vi "Save Data_IIT.vi"(0 "Experiment Indicator":string, 3 "Scan direction":i32, 4 "Data Array":dbl[][](array[numeric]), 6 "Username":string, 7 "Stabilisation time (ms)":dbl, 8 "Cell details cluster":T1={"Cell Position"=16, "Cell Label"="", "Pixel to measure"=0, "Area (cm^2)"=0.126, "Variable"="", "Variable value"="", "Scan settings in queue"=0, "Light or dark"="", "Measurement Type"=""} {"Pixel to measure" items=["All", "1", "2", "3", "4", "5", "6", "7", "8"]}, 10 "Measurement Delay (ms)":dbl=1.0, 11 "Stabilisation level \n(A or V depending on mode)":dbl=-1.4, 13 "Stabilisation Data":dbl[][](array[numeric])) -> (14 "Master Log":string[][](table), 15 "File path for master log":path, 17 "File path for JV data":path, 18 "File path for JV image":path)   [LabVIEW 2011]
uses:
  <vilib>/Utility/file.llb/Write To Spreadsheet File (string).vi
  <vilib>/Utility/file.llb/Read From Spreadsheet File (string).vi
  <vilib>/Analysis/NI_AALPro.lvlib
panel:
  out "Vmp":dbl
  out "PCE":dbl
  out "FF":dbl
  out "Voc":dbl
  out "Jsc":dbl
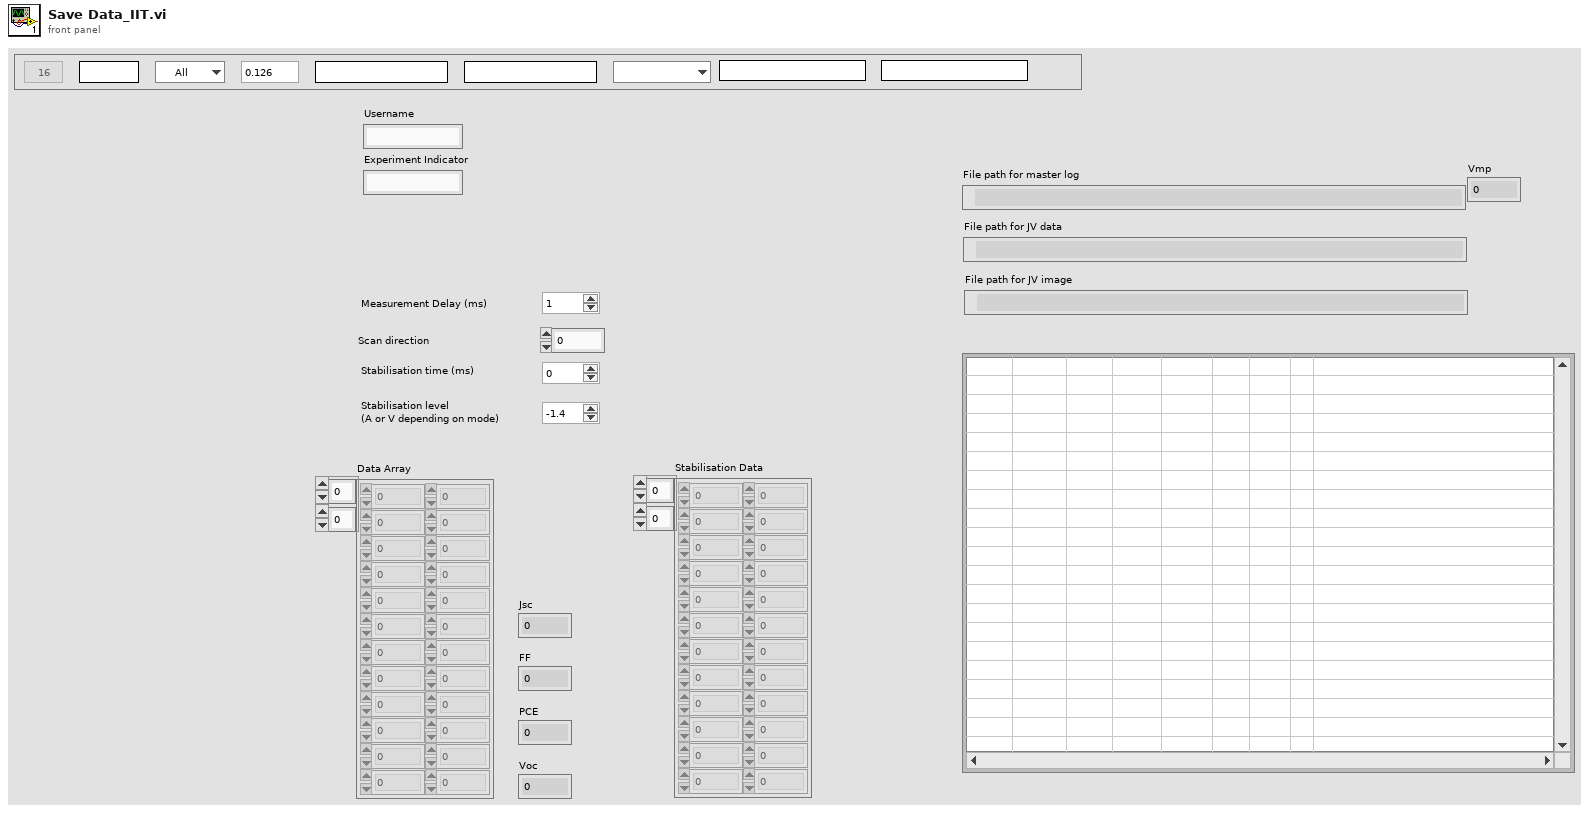
[diagram p1: front panel]
types:
  T1 = cluster{"Cell Position":i32, "Cell Label":string, "Pixel to measure":u16, "Area (cm^2)":dbl, "Variable":string, "Variable value":string, "Scan settings in queue":u16, "Light or dark":string, "Measurement Type":string}
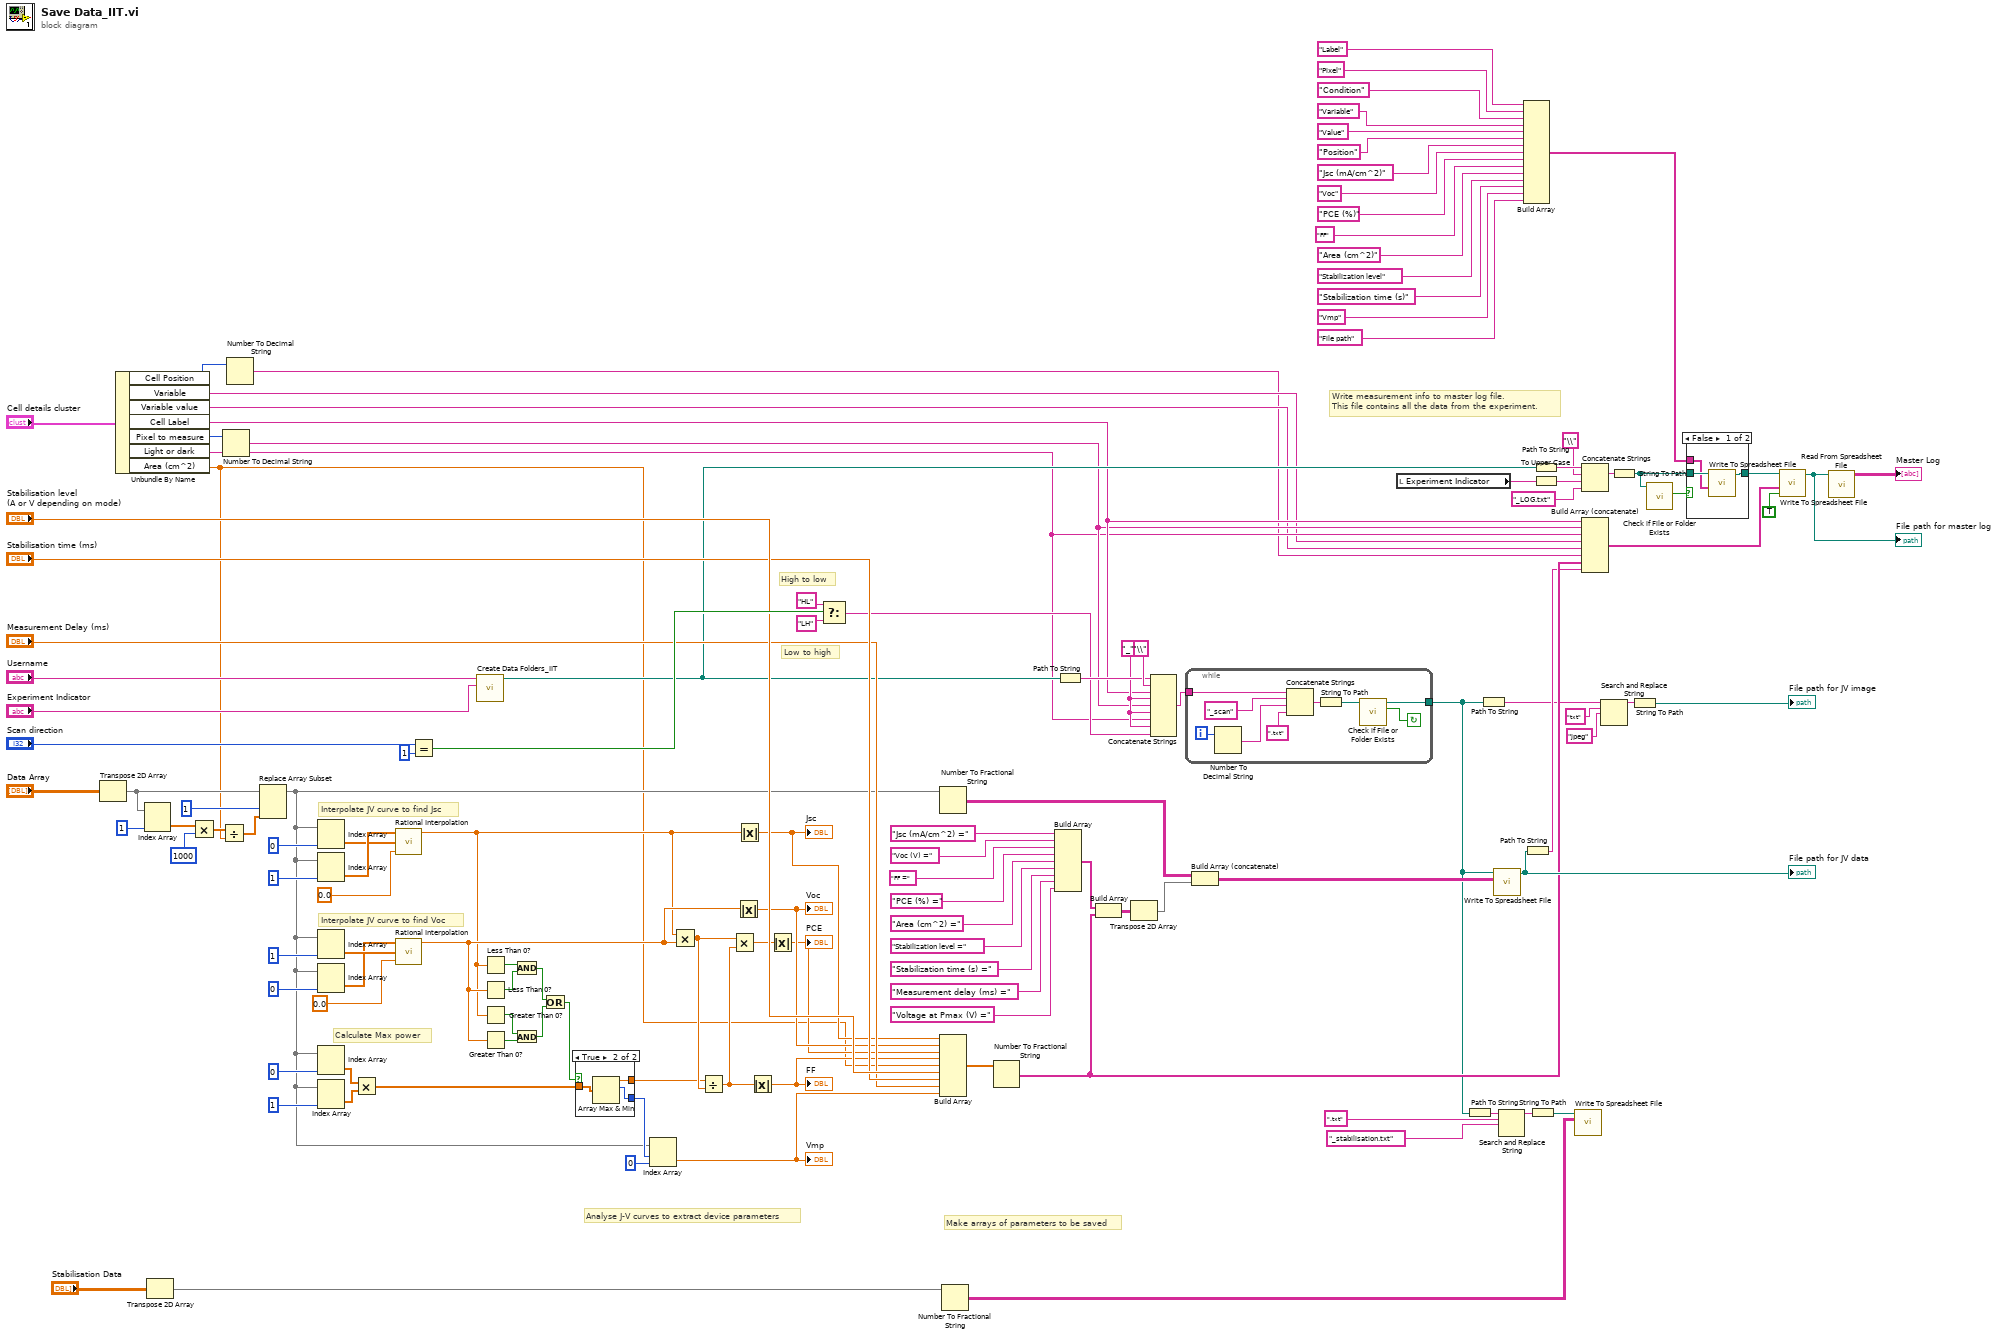
[diagram p0: block diagram]
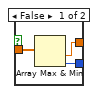
[diagram p3: hidden frame]
diagram:
  w45 = "_"
  # "Make arrays of parameters to be saved"
  # "Calculate Max power"
  # "Interpolate JV curve to find Voc"
  # "Interpolate JV curve to find Jsc"
  # "Analyse J-V curves to extract device parameters"
  # "Write measurement info to master log file.\nThis file contains all the data from the experiment."
  # "Low to high"
  # "High to low"
  n1 = Transpose 2D Array(2D array="Data Array") -> (transposed array=w53:dbl[][])
  n2 = Unbundle By Name("Cell details cluster") -> ("Cell Position"=w26:i32, "Variable"=w22:string, "Variable value"=w21:string, "Cell Label"=w25:string, "Pixel to measure"=w27:u16, "Light or dark"=w23:string, "Area (cm^2)"=w28:dbl)
  n3 = Index Array(array=w53, index (col)=1) -> (element=w51:dbl[])  [unwired: 1 in]
  n4 = Transpose 2D Array(2D array="Stabilisation Data") -> (transposed array=w35:dbl[][])
  n5 = Multiply(x=w51, y=1000) -> (x*y=w48:dbl[])
  n6 = Divide(x=w48, y=w28) -> (x/y=w47:dbl[])
  n7 = Number To Decimal String(number=w27) -> (decimal integer string=w24:string)  [unwired: 1 in]
  n8 = Number To Decimal String(number=w26) -> (decimal integer string=w20:string)  [unwired: 1 in]
  n9 = Replace Array Subset(array=w53, new element=w47, index (col)=1) -> (w32:dbl[][])  [unwired: 1 in]
  n10 = Index Array(array=w32, index (col)=0) -> (element=w120:dbl[])  [unwired: 1 in]
  n11 = Index Array(array=w32, index (col)=1) -> (element=w121:dbl[])  [unwired: 1 in]
  n12 = Index Array(array=w32, index (col)=1) -> (element=w119:dbl[])  [unwired: 1 in]
  n13 = Index Array(array=w32, index (col)=0) -> (element=w117:dbl[])  [unwired: 1 in]
  n14 = Index Array(array=w32, index (col)=0) -> (element=w125:dbl[])  [unwired: 1 in]
  n15 = Index Array(array=w32, index (col)=1) -> (element=w124:dbl[])  [unwired: 1 in]
  n16 = Multiply(x=w125, y=w124) -> (x*y=w118:dbl[])
  n17 = call <vilib>:"Rational Interpolation.vi"("x value"=0.0, "X"=w120, "Y"=w121) -> ("interpolation value"=w49:dbl)  [unwired: 2 out]
  n18 = call <vilib>:"Rational Interpolation.vi"("x value"=0.0, "X"=w119, "Y"=w117) -> ("interpolation value"=w60:dbl)  [unwired: 2 out]
  n19 = Equal?(x="Scan direction", y=1) -> (x = y?=w84:bool)
  n20 = call "Create Data Folders_IIT.vi"("Experiment Indicator"="Experiment Indicator", "username"="Username") -> ("Data Output Folder"=w75:path)  [unwired: 9 in]
  n21 = Less Than 0?(x=w49) -> (x < 0?=w66:bool)
  n22 = Less Than 0?(x=w60) -> (x < 0?=w63:bool)
  n23 = Greater Than 0?(x=w49) -> (x > 0?=w64:bool)
  n24 = Greater Than 0?(x=w60) -> (x > 0?=w65:bool)
  n25 = And(x=w66, y=w63) -> (x .and. y?=w68:bool)
  n26 = And(x=w64, y=w65) -> (x .and. y?=w67:bool)
  n27 = Or(x=w68, y=w67) -> (x .or. y?=w62:bool)
  n28 = case shown="True" w62 {
    tunnel: [w133 w137] -> w46
    tunnel: w118 -> [w134 w136]
    tunnel: [w132 w135] -> w33
    frame False {
      n29 = Array Max & Min(array=w134) -> (min value=w133:dbl, min index (indices)=w132:i32)  [unwired: 2 out]
    }
    frame True {
      n30 = Array Max & Min(array=w136) -> (max value=w137:dbl, max index (indices)=w135:i32)  [unwired: 2 out]
    }
  }
  n31 = Index Array(array=w32, index (row)=w33, index (col)=0) -> (element=w30:dbl)
  "Vmp" <- w30
  n32 = Multiply(x=w49, y=w60) -> (x*y=w116:dbl)
  n33 = Divide(x=w46, y=w116) -> (x/y=w56:dbl)
  n34 = Multiply(x=w116, y=w56) -> (x*y=w58:dbl)
  n35 = Absolute Value(x=w60) -> (abs(x)=w59:dbl)
  "Voc" <- w59
  n36 = Absolute Value(x=w49) -> (abs(x)=w61:dbl)
  "Jsc" <- w61
  n37 = Absolute Value(x=w56) -> (abs(x)=w55:dbl)
  "FF" <- w55
  n38 = Absolute Value(x=w58) -> (abs(x)=w57:dbl)
  "PCE" <- w57
  n39 = Select(t="HL", s=w84, f="LH") -> (s? t:f=w44:string)
  n40 = Number To Fractional String(number=w32) -> (F-format string=w86:string[][])  [unwired: 3 in]
  n41 = Build Array(w61, w59, w57, w55, w28, "Stabilisation level \n(A or V depending on mode)", "Stabilisation time (ms)", "Measurement Delay (ms)", w30) -> (w111:dbl[])
  n42 = Number To Fractional String(number=w35) -> (F-format string=w36:string[][])  [unwired: 3 in]
  n43 = Number To Fractional String(number=w111) -> (F-format string=w76:string[])  [unwired: 3 in]
  n44 = Build Array("Jsc (mA/cm^2) =", "Voc (V) =", "FF =", "PCE (%) =", "Area (cm^2) =", "Stabilization level =", "Stabilization time (s) =", "Measurement delay (ms) =", "Voltage at Pmax (V) =") -> (w110:string[])
  n45 = Path To String(path=w75) -> (string=w95:string)
  n46 = Build Array(w110, w76) -> (w106:string[][])
  n47 = Transpose 2D Array(2D array=w106) -> (transposed array=w105:string[][])
  n48 = Concatenate Strings(w95, "\\", w25, w45, w24, w45, w23, w45, w44) -> (w73:string)
  n49 = while {
    tunnel: w73 -> [w146]
    tunnel: [w138] -> w42
    i -> [w144]
    stop <- w139 continue-if-true
    n50 = Number To Decimal String(number=w144) -> (decimal integer string=w143:string)  [unwired: 1 in]
    n51 = Concatenate Strings(w146, "_scan", w143, ".txt") -> (w140:string)
    n52 = String To Path(string=w140) -> (path=w141:path)
    n53 = call <vilib>:"Check if File or Folder Exists.vi"("path"=w141) -> ("file or folder exists?"=w139:bool, "dup path"=w138:path)  [unwired: 8 in, 1 out]
  }
  n54 = Build Array (concatenate)(w86, w105) -> (w109:string[][])
  n55 = local read "Experiment Indicator"() -> (w69:string)
  n56 = Path To String(path=w42) -> (string=w41:string)
  n57 = Path To String(path=w42) -> (string=w72:string)
  n58 = call-poly <vilib>:"Write To Spreadsheet File.vi"("2D data"=w109, "file path (dialog if empty)"=w42) -> ("new file path (Not A Path if cancelled)"=w82:path)  [unwired: 6 in]
  "File path for JV data" <- w82
  n59 = Search and Replace String(input string=w41, search string=".txt", replace string="_stabilisation.txt") -> (result string=w38:string)  [unwired: 5 in, 3 out]
  n60 = Build Array("Label", "Pixel", "Condition", "Variable", "Value", "Position", "Jsc (mA/cm^2)", "Voc", "PCE (%)", "FF", "Area (cm^2)", "Stabilization level", "Stabilization time (s)", "Vmp", "File path") -> (w1:string[])
  n61 = Path To String(path=w82) -> (string=w74:string)
  n62 = String To Path(string=w38) -> (path=w37:path)
  n63 = Path To String(path=w75) -> (string=w101:string)
  n64 = To Upper Case(1:w69) -> (0:w70:string)
  n65 = call-poly <vilib>:"Write To Spreadsheet File.vi"("2D data"=w36, "file path (dialog if empty)"=w37) -> ()  [unwired: 6 in, 1 out]
  n66 = Concatenate Strings(w101, "\\", w70, "_LOG.txt") -> (w99:string)
  n67 = Build Array (concatenate)(w25, w24, w23, w22, w21, w20, w76, w74) -> (w98:string[])
  n68 = Search and Replace String(input string=w72, search string="txt", replace string="jpeg") -> (result string=w94:string)  [unwired: 5 in, 3 out]
  n69 = String To Path(string=w99) -> (path=w3:path)
  n70 = String To Path(string=w94) -> (path=→"File path for JV image":path)
  n71 = call <vilib>:"Check if File or Folder Exists.vi"("path"=w3) -> ("file or folder exists?"=w4:bool)  [unwired: 8 in, 2 out]
  n72 = case shown="False" w4 {
    tunnel: w3 -> [w149 w150]
    tunnel: [w148 w150] -> w2
    tunnel: w1 -> [w147 _]
    frame False {
      n73 = call-poly <vilib>:"Write To Spreadsheet File.vi"("1D data"=w147, "file path (dialog if empty)"=w149) -> ("new file path (Not A Path if cancelled)"=w148:path)  [unwired: 6 in]
    }
    frame True {
    }
  }
  n74 = call-poly <vilib>:"Write To Spreadsheet File.vi"("append to file? (new file:F)"=TRUE, "1D data"=w98, "file path (dialog if empty)"=w2) -> ("new file path (Not A Path if cancelled)"=w89:path)  [unwired: 5 in]
  "File path for master log" <- w89
  n75 = call-poly <vilib>:"Read From Spreadsheet File.vi"("file path (dialog if empty)"=w89) -> ("all rows"=→"Master Log":string[][])  [unwired: 6 in, 4 out]
